vi "Reset.vi"(8 "error in (no error)":errorcluster, 11 "Proto Tag in":refnum<class "packed.lvclass">) -> (0 "error out":errorcluster, 3 "Proto Tag out":refnum<class "packed.lvclass">)   [LabVIEW 2020, in "Protobuf RAW.lvlib" / "packed.lvclass"]
uses:
  packed.lvclass
  packed.lvclass/packed.ctl
  Scalar Encoder/Scalar Type.lvclass
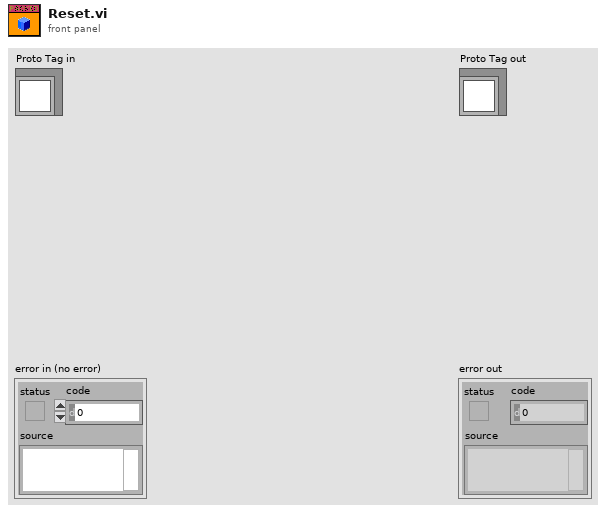
[diagram p1: front panel]
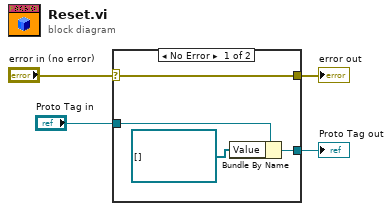
[diagram p0: block diagram]
diagram:
  n1 = case shown="No Error" "error in (no error)" {
    selector: "error in (no error)" -> [w6 w10]
    tunnel: "Proto Tag in" -> [w8 w9]
    tunnel: [w5 w9] -> w1
    tunnel: [w6 w10] -> w2
    frame No Error {
      n2 = Bundle By Name(cluster=w8, "Value"=refnum<class "Scalar Type.lvclass">[] []) -> (w5:refnum<class "packed.lvclass">)
    }
    frame Error {
    }
  }
  "error out" <- w2
  "Proto Tag out" <- w1
